vi "Send New Job.vi"(8 "error in (no error)":errorcluster, 9 "Build":string, 10 "Max Progress":i32, 11 "Build Events API in":refnum<class "Build Events API.lvclass">) -> (0 "error out":errorcluster, 3 "Build Events API out":refnum<class "Build Events API.lvclass">)   [LabVIEW 2020, in "Builder Tools.lvlib" / "Build Events API.lvclass"]
uses:
  Build Events API.lvclass
  New Job Data.ctl
  Build Events API.lvclass/Build Events API.ctl
  Builder Tools.lvlib
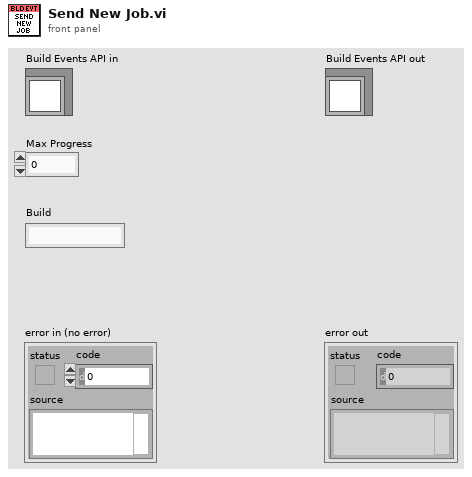
[diagram p1: front panel]
types:
  T1 = typedef "Builder Tools.lvlib/New Job Data.ctl" = cluster{"Max Progress":i32, "Build":string}
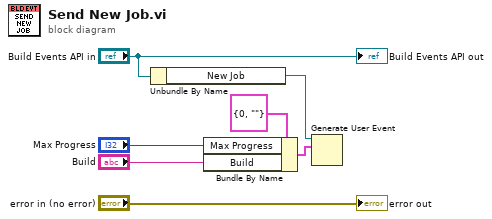
[diagram p0: block diagram]
diagram:
  n1 = Unbundle By Name("Build Events API in") -> ("New Job"=w5:refnum<user-event>)
  n2 = Bundle By Name(cluster=T1 {"Max Progress"=0, "Build"=""} ("event data"), "Max Progress"="Max Progress", "Build"="Build") -> (w3:T1)
  n3 = Generate User Event(user event=w5, event data cluster=w3) -> ()  [unwired: 2 in, 2 out]
  "error out" <- "error in (no error)"
  "Build Events API out" <- "Build Events API in"
